vi "Command Write.vi"(1 "Path":path, 3 "error in (no error)":errorcluster) -> (10 "error out":errorcluster)   [LabVIEW 2017]
uses:
  <vilib>/Utility/file.llb/Write Delimited Spreadsheet (string).vi
panel:
  in  "Command Data 2":dbl[](array[numeric])
  in  "Command Data":dbl[](array[numeric])
  in  "Command Name":string[](array[combo])
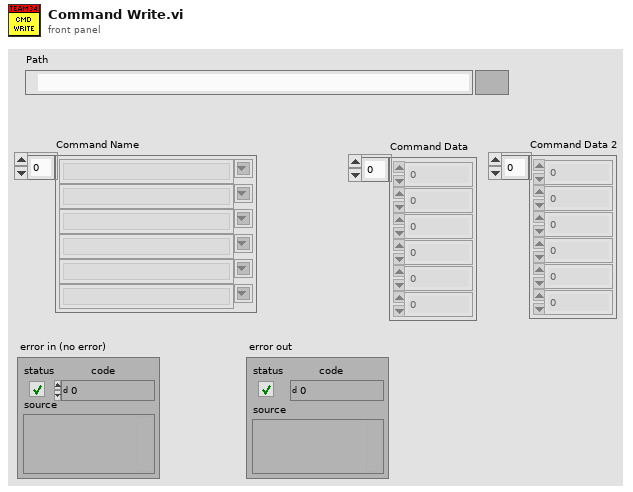
[diagram p1: front panel]
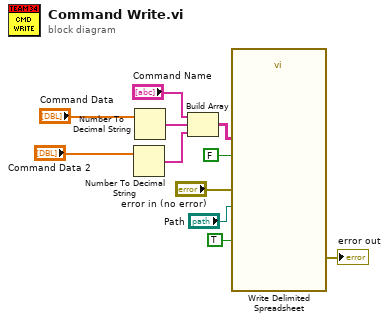
[diagram p0: block diagram]
diagram:
  n1 = Number To Decimal String(number="Command Data 2") -> (decimal integer string=w2:string[])  [unwired: 1 in]
  n2 = Number To Decimal String(number="Command Data") -> (decimal integer string=w5:string[])  [unwired: 1 in]
  n3 = Build Array("Command Name", w5, w2) -> (w7:string[][])
  n4 = call-poly <vilib>:"Write Delimited Spreadsheet.vi"("file path (dialog if empty)"="Path", "2D data"=w7, "append to file? (new file:F)"=FALSE, "error in (no error)"="error in (no error)", "transpose? (no:F)"=TRUE) -> ("error out"=→"error out":errorcluster)  [unwired: 9 in, 1 out]
